vi "QAM Modulation.vi"(10 "pulse shaping filter (none)":T1(ring), 11 "coerced IQ rate":dbl) -> (2 "output complex waveform":T2 {"Y" format="%.3f"; "dt" format="%^.2e"; "t0" format="%.4f"}, 3 "output bit stream":i8[](array[numeric]))   [LabVIEW 2026]
uses:
  <vilib>/addons/Modulation/Analog/controls/Complex Data Waveform.ctl
  <vilib>/addons/Modulation/Digital/General/MT Generate Bits (Galois, PN Order).vi
  <vilib>/addons/Modulation/Digital/Support/Common/Validators/mod_Generate Bits Validate.vi
  <vilib>/addons/Modulation/Analog/support/mod_Set Error Source.vi
  <vilib>/addons/Modulation/Analog/support/Validators/mod_Fractional Resample Validate.vi
  <vilib>/addons/Modulation/Analog/support/Validators/mod_Check Flush State.vi
  <vilib>/addons/Modulation/Analog/support/mod_FractionalResampler.vi
  <vilib>/addons/Modulation/Analog/support/mod_Integer Rate Interpolation.vi
  <vilib>/addons/Modulation/Analog/support/Validators/mod_Validate Complex Waveform.vi
  <vilib>/addons/Modulation/Analog/support/mod_PerformResampling.vi
  <vilib>/addons/Modulation/Analog/support/Validators/mod_WFErrorHandler.vi
  <vilib>/addons/Modulation/Digital/General/MT Generate QAM System Parameters(M).vi
  <vilib>/addons/Modulation/Digital/General/subVIs/mod_Generate Bits PN Sequence.vi
  <vilib>/addons/Modulation/Digital/Support/Common/Validators/mod_Generate Filter Coefficients Validate.vi
  <vilib>/addons/Modulation/Digital/General/subVIs/mod_Generate Filter Coefficients.vi
  <vilib>/Utility/error.llb/Error Cluster From Error Code.vi
  <vilib>/addons/Modulation/Analog/support/mod_Resampling Factors.vi
  <vilib>/addons/Modulation/Analog/support/mod_ResamplingFilter.vi
  <vilib>/addons/Modulation/Analog/support/mod_Generate Integer Interpolation Filter.vi
  <vilib>/addons/Modulation/niDMT.lvlib
  <vilib>/addons/Modulation/niAMT.lvlib
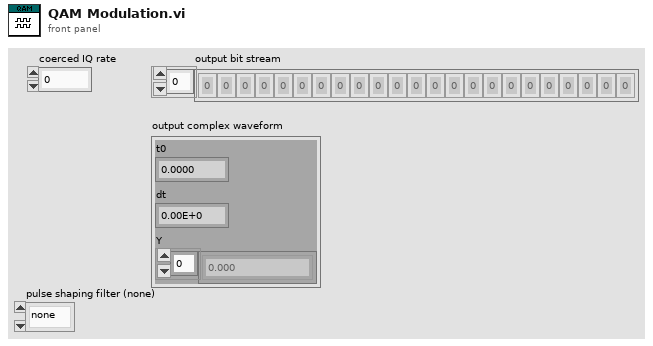
[diagram p1: front panel]
types:
  T1 = enum16{"none", "Raised Cosine", "Root Raised Cos", "Gaussian"}
  T2 = typedef "niAMT.lvlib/Complex Data Waveform.ctl" = cluster{"t0":dbl, "dt":dbl, "Y":cdb[]}
  T3 = enum16{"FSK", "PSK", "QAM", "MSK", "PAM", "ASK", "CPM"}
  T4 = cluster{"samples per symbol (16)":i32, "symbol map":cdb[]}
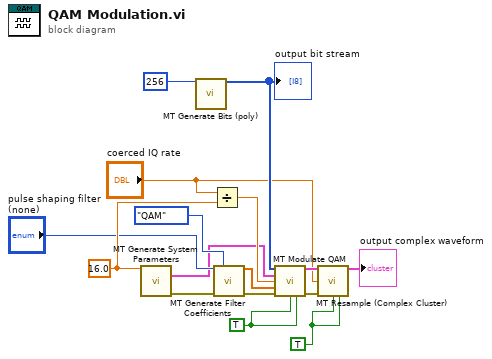
[diagram p0: block diagram]
diagram:
  w15 = TRUE ("reset? (T)")
  w16 = 16.0 ("y")
  w6 = TRUE ("reset? (T)")
  n1 = call-poly <vilib>:"MT Generate System Parameters.vi"("samples per symbol (16)"=w16) -> ("QAM system parameters"=w8:T4, "error out"=w11:errorcluster)  [unwired: 12 in, 1 out]
  n2 = call-poly <vilib>:"MT Generate Bits (poly).vi"("total bits (128)"=256) -> ("output bit stream"=w3:i8[])  [unwired: 12 in, 2 out]
  "output bit stream" <- w3
  n3 = Divide(x="coerced IQ rate", y=w16) -> (x/y=w12:dbl)
  n4 = call <vilib>:"MT Generate Filter Coefficients.vi"("pulse shaping filter (none)"="pulse shaping filter (none)", "modulation type"=T3."QAM", "error in (no error)"=w11) -> ("pulse shaping filter coefficients"=w7:dbl[], "error out"=w10:errorcluster)  [unwired: 10 in, 1 out]
  n5 = call <vilib>:"MT Modulate QAM.vi"("input bit stream"=w3, "QAM system parameters"=w8, "symbol rate (Hz)"=w12, "pulse shaping filter coefficients"=w7, "error in (no error)"=w10, "reset? (T)"=w15, "flush buffers? (F)"=w15) -> ("output complex waveform"=w4:T2, "error out"=w5:errorcluster)  [unwired: 6 in, 1 out]
  n6 = call <vilib>:"MT Resample (Complex Cluster).vi"("input complex waveform"=w4, "desired sample rate (Hz)"="coerced IQ rate", "error in (no error)"=w5, "reset? (T)"=w6, "flush buffers? (F)"=w6) -> ("output complex waveform"=→"output complex waveform":T2)  [unwired: 9 in, 1 out]
